vi "Initialize.vi"(0 "Moving Ripple Noise in":refnum<class "Moving Ripple Noise.lvclass">, 1 "Filter in":refnum<class "Filter.lvclass">, 5 "Level in":refnum<class "Level.lvclass">, 7 "Fs (Hz)":dbl, 9 "Npts":i32, 11 "error in (no error)":errorcluster, 13 "Channel Name":string) -> (3 "Filter out":refnum<class "Filter.lvclass">, 4 "Moving Ripple Noise out":refnum<class "Moving Ripple Noise.lvclass">, 6 "Level out":refnum<class "Level.lvclass">, 15 "error out":errorcluster)   [LabVIEW 2020, in "Moving Ripple Noise.lvclass"]
uses:
  Moving Ripple Noise.lvclass
  Level/Level.lvclass
  Filter/Filter.lvclass
  Moving Ripple Noise.lvclass/Moving Ripple Noise.ctl
  Utility VIs/Math VIs/LinSpace (x0-dx-npts).vi
  <vilib>/Analysis/NI_AALBase.lvlib
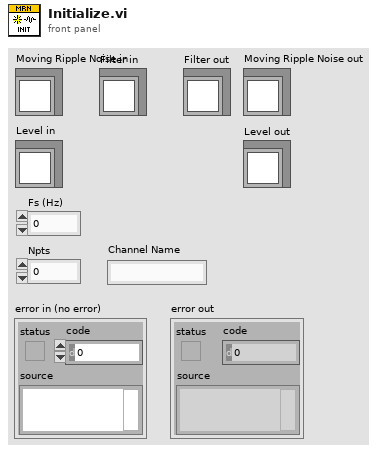
[diagram p1: front panel]
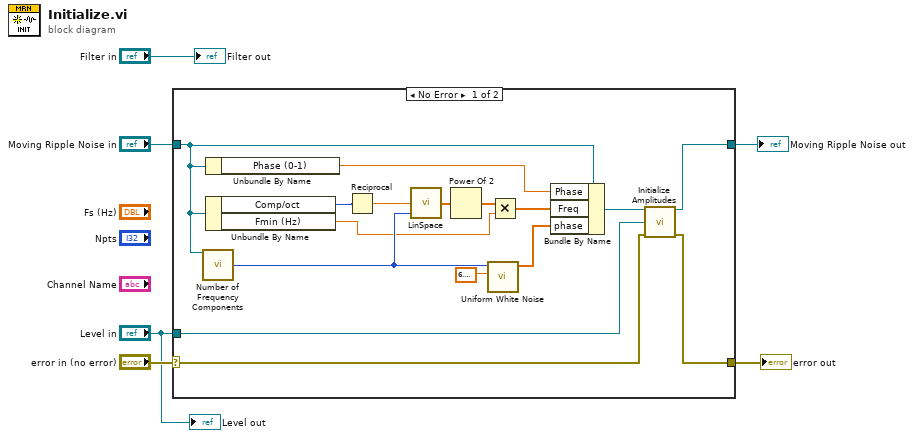
[diagram p0: block diagram]
diagram:
  n1 = case shown="No Error" "error in (no error)" {
    selector: "error in (no error)" -> [w13 w23]
    tunnel: [w12 w24] -> w4
    tunnel: "Moving Ripple Noise in" -> [w9 w24]
    tunnel: [w11 w23] -> w2
    tunnel: "Level in" -> [w10 _]
    frame No Error {
      n2 = call "Number of Frequency Components.vi"("MRN in"=w9) -> ("Nfreq"=w8:i32)  [unwired: 12 in, 2 out]
      n3 = Unbundle By Name(w9) -> ("Phase (0-1)"=w15:dbl)
      n4 = Unbundle By Name(w9) -> ("Comp/oct"=w22:i32, "Fmin (Hz)"=w7:dbl)
      n5 = Reciprocal(x=w22) -> (1/x=w18:dbl)
      n6 = call-poly "LinSpace.vi"("npts"=w8, "dx"=w18) -> ("Array"=w19:dbl[])  [unwired: 2 in, 1 out]
      n7 = Power Of 2(x=w19) -> (2^x=w20:dbl[])
      n8 = call <vilib>:"Uniform White Noise.vi"("amplitude"=6.283185307179586, "samples"=w8) -> ("uniform white noise"=w16:dbl[])  [unwired: 8 in, 1 out]
      n9 = Multiply(x=w20, y=w7) -> (x*y=w17:dbl[])
      n10 = Bundle By Name(cluster=w9, "Phase"=w15, "Freq"=w17, "phase"=w16) -> (w14:refnum<class "Moving Ripple Noise.lvclass">)
      n11 = call "Initialize Amplitudes.vi"("MRN in"=w14, "Level in"=w10, "error in (no error)"=w13) -> ("MRN out"=w12:refnum<class "Moving Ripple Noise.lvclass">, "error out"=w11:errorcluster)  [unwired: 11 in]
    }
    frame Error {
    }
  }
  "error out" <- w2
  "Moving Ripple Noise out" <- w4
  "Level out" <- "Level in"
  "Filter out" <- "Filter in"
